vi "Get Plugin Paths.vi"(0 "MeasurementService in":refnum<class "MeasurementPluginService.lvclass">, 11 "error in (no error)":errorcluster) -> (4 "MeasurementService out":refnum<class "MeasurementPluginService.lvclass">, 6 "Get Measurement Details VI Path":path, 8 "Measurement Logic VI Path":path, 10 "Measurement UI VI Path":path, 13 "Measurement Configuration CTL Path":path, 14 "Measurement Results CTL Path":path, 15 "error out":errorcluster)   [LabVIEW 2020, in "MeasurementLink Measurement Server.lvlib" / "MeasurementPluginService.lvclass"]
uses:
  MeasurementPluginService.lvclass
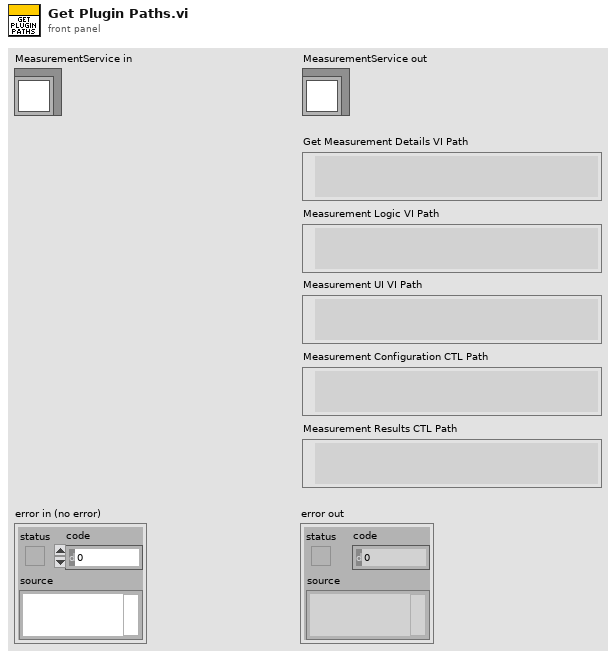
[diagram p1: front panel]
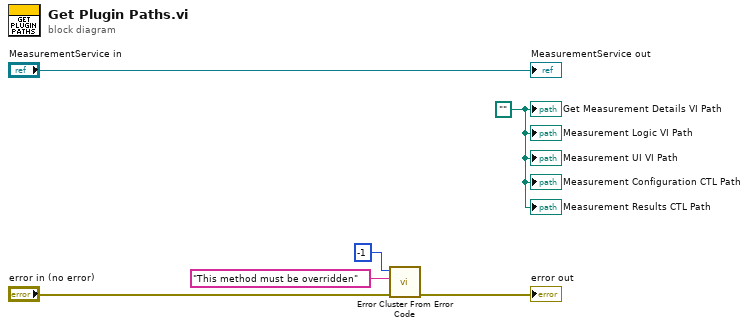
[diagram p0: block diagram]
diagram:
  w1 = path ""
  n1 = call <vilib>:"Error Cluster From Error Code.vi"("error in (no error)"="error in (no error)", "error message (\"\")"="This method must be overridden" ("error message (\"\")"), "error code (0)"=-1) -> ("error out"=→"error out":errorcluster)  [unwired: 6 in]
  "MeasurementService out" <- "MeasurementService in"
  "Measurement Results CTL Path" <- w1
  "Get Measurement Details VI Path" <- w1
  "Measurement Logic VI Path" <- w1
  "Measurement UI VI Path" <- w1
  "Measurement Configuration CTL Path" <- w1
